vi "line_initialise_image.vi"(8 "error in (no error)":errorcluster, 11 "AnalysisRAPS in":refnum<class "AnalysisRAPS.lvclass">) -> (0 "error out":errorcluster, 3 "AnalysisRAPS out":refnum<class "AnalysisRAPS.lvclass">)   [LabVIEW 2010, in "AnalysisRAPS.lvclass"]
uses:
  AnalysisRAPS.lvclass
  AnalysisRAPS.lvclass/AnalysisRAPS.ctl
  common/libraries/TIFFManagement/TIFFManagement.lvlib
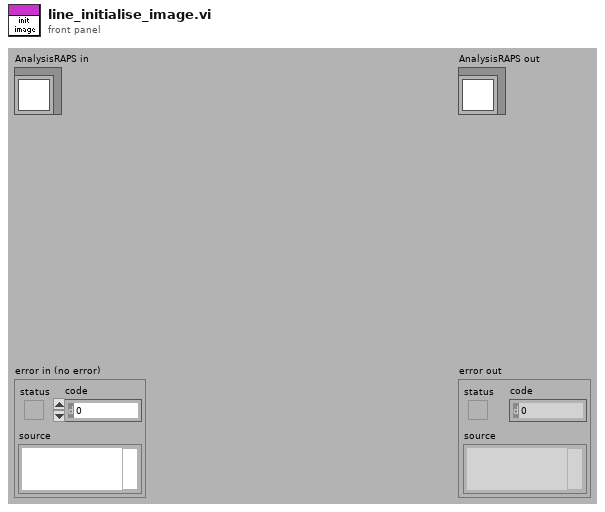
[diagram p1: front panel]
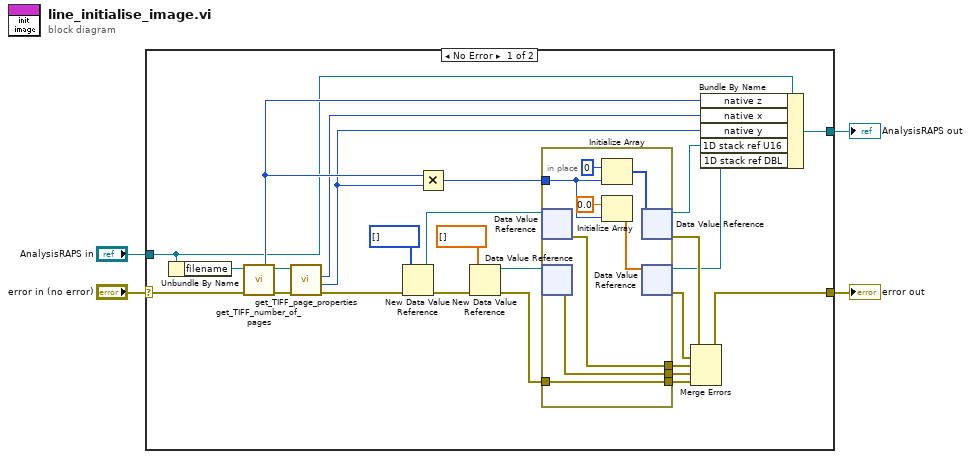
[diagram p0: block diagram]
diagram:
  n1 = case shown="No Error" "error in (no error)" {
    selector: "error in (no error)" -> [w21 w39]
    tunnel: [w10 w39] -> w3
    tunnel: [w26 w38] -> w1
    tunnel: "AnalysisRAPS in" -> [w19 w38]
    frame No Error {
      n2 = Unbundle By Name(w19) -> ("filename"=w22:path)
      n3 = call "get_TIFF_number_of_pages.vi"("error in (no error)"=w21, "path in"=w22) -> ("error out"=w16:errorcluster, "number of pages"=w20:i32, "path out"=w17:path)  [unwired: 7 in]
      n4 = call "get_TIFF_page_properties.vi"("error in (no error)"=w16, "path in"=w17) -> ("error out"=w15:errorcluster, "height"=w14:i32, "width"=w18:i32)  [unwired: 3 in, 4 out]
      n5 = New Data Value Reference(data value=u16[] [], error in=w15) -> (data value reference=w28:refnum<data-value>, error out=w13:errorcluster)
      n6 = Multiply(x=w20, y=w14) -> (x*y=w25:i32)
      n7 = New Data Value Reference(data value=dbl[] [], error in=w13) -> (data value reference=w11:refnum<data-value>, error out=w12:errorcluster)
      n8 = in-place {
        in-place-border: [w37] -> w27
        in-place-border: w25 -> [w30]
        in-place-border: [w34] -> w24
        in-place-border: w12 -> [w33]
        in-place-border: [w33] -> w8
        n9 = in-place-dvr #1(w28) -> (w37:errorcluster)  [unwired: 1 out]
        n10 = in-place-dvr #2(w11) -> (w34:errorcluster)  [unwired: 1 out]
        n11 = Initialize Array(u16 0, w30) -> (w35:u16[])
        n12 = Initialize Array(0.0 ("element"), w30) -> (w31:dbl[])
        n13 = in-place-dvr #1(w35) -> (w23:refnum<data-value>, w7:errorcluster)
        n14 = in-place-dvr #2(w31) -> (w5:refnum<data-value>, w6:errorcluster)
      }
      n15 = Merge Errors(w7, w6, w27, w24, w8) -> (w10:errorcluster)
      n16 = Bundle By Name(cluster=w19, "native z"=w20, "native x"=w18, "native y"=w14, "1D stack ref U16"=w23, "1D stack ref DBL"=w5) -> (w26:refnum<class "AnalysisRAPS.lvclass">)
    }
    frame Error {
    }
  }
  "error out" <- w3
  "AnalysisRAPS out" <- w1
